vi "ep_Input Power Method.vi"(6 "total input active power [W]":dbl, 8 "error in (no error)":errorcluster, 9 "nameplate information":T1, 11 "efficiency values [%]":dbl[](array[numeric])) -> (0 "error out":errorcluster, 2 "efficiency [%]":dbl, 3 "load [W]":dbl)   [LabVIEW 2014, in "NI_EP_Motor Monitoring.lvlib"]
uses:
  <vilib>/addons/Electrical Power/Motor Monitoring/NI_EP_Motor Monitoring.lvlib
  <vilib>/addons/Electrical Power/Motor Monitoring/subVIs/ep_Input Power Algorithm.ctl
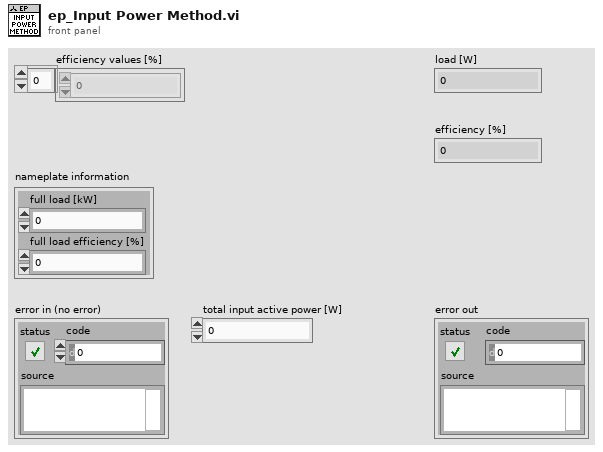
[diagram p1: front panel]
types:
  T1 = cluster{"full load [kW]":dbl, "full load efficiency [%]":dbl}
  T2 = typedef "NI_EP_Motor Monitoring.lvlib/ep_Input Power Algorithm.ctl" = enum16{"interpolate eff.", "use min eff.", "use default eff."}
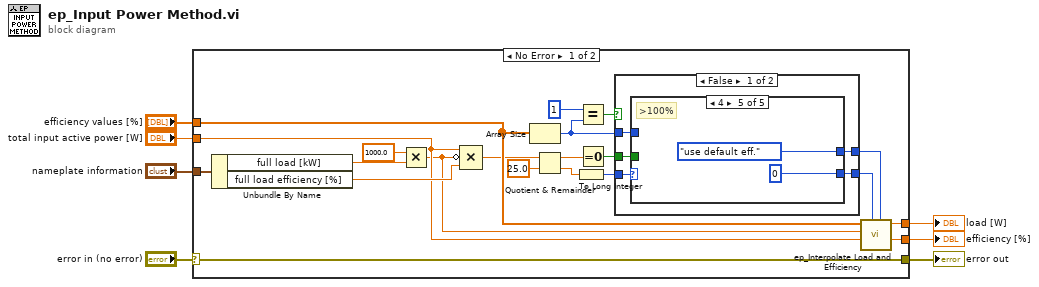
[diagram p0: block diagram]
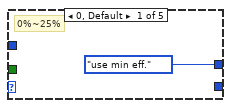
[diagram p2: hidden frame]
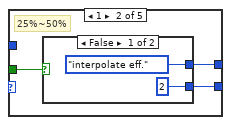
[diagram p3: hidden frame]
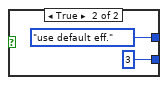
[diagram p4: hidden frame]
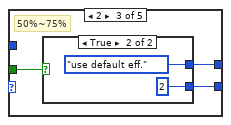
[diagram p5: hidden frame]
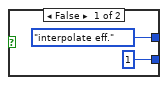
[diagram p6: hidden frame]
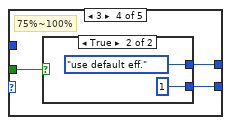
[diagram p7: hidden frame]
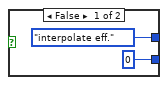
[diagram p8: hidden frame]
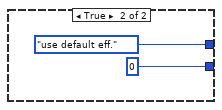
[diagram p9: hidden frame]
diagram:
  n1 = case shown="No Error" "error in (no error)" {
    selector: "error in (no error)" -> [w28 w60]
    tunnel: "efficiency values [%]" -> [w20 _]
    tunnel: "nameplate information" -> [w27 _]
    tunnel: "total input active power [W]" -> [w12 _]
    tunnel: [w28 w60] -> w3
    tunnel: [w26 _] -> w2
    tunnel: [w11 _] -> w1
    frame No Error {
      n2 = Unbundle By Name(w27) -> ("full load [kW]"=w9:dbl, "full load efficiency [%]"=w19:dbl)
      n3 = Multiply(x=1000.0, y=w9) -> (x*y=w10:dbl)
      n4 = Compound Arithmetic op=MULTIPLY(w12, invert w10, w19) -> (w15:dbl)
      n5 = Array Size(array=w20) -> (size(s)=w23:i32)
      n6 = Quotient & Remainder(x=w15, y=25.0) -> (x-y*floor(x/y)=w14:dbl, floor(x/y)=w17:dbl)
      n7 = To Long Integer(number=w17) -> (32bit integer=w25:i32)
      n8 = Equal?(x=1, y=w23) -> (x = y?=w24:bool)
      n9 = Equal To 0?(x=w14) -> (x = 0?=w13:bool)
      n10 = case shown="False" w24 {
        tunnel: w25 -> [w33 _]
        tunnel: [w32 ep_Input_Power_Algorithm."use default eff." ("algorithm")] -> w21
        tunnel: [w31 0] -> w22
        tunnel: w23 -> [w30 _]
        tunnel: w13 -> [w29 _]
        frame False {
          n11 = case shown="4" w33 {
            tunnel: [ep_Input_Power_Algorithm."use min eff." ("algorithm") w37 w44 w51 ep_Input_Power_Algorithm."use default eff." ("algorithm")] -> w32
            tunnel: [_ w36 w43 w50 0] -> w31
            tunnel: w30 -> [_ _ _ _ _]
            tunnel: w29 -> [_ w35 w42 w49 _]
            frame 0, Default {
              # "0%~25%"
            }
            frame 1 {
              # "25%~50%"
              n12 = case shown="False" w35 {
                tunnel: [ep_Input_Power_Algorithm."interpolate eff." ("algorithm") ep_Input_Power_Algorithm."use default eff." ("algorithm")] -> w37
                tunnel: [2 3] -> w36
                frame False {
                }
                frame True {
                }
              }
            }
            frame 2 {
              # "50%~75%"
              n13 = case shown="True" w42 {
                tunnel: [ep_Input_Power_Algorithm."interpolate eff." ("algorithm") ep_Input_Power_Algorithm."use default eff." ("algorithm")] -> w44
                tunnel: [1 2] -> w43
                frame False {
                }
                frame True {
                }
              }
            }
            frame 3 {
              # "75%~100%"
              n14 = case shown="True" w49 {
                tunnel: [ep_Input_Power_Algorithm."interpolate eff." ("algorithm") ep_Input_Power_Algorithm."use default eff." ("algorithm")] -> w51
                tunnel: [0 1] -> w50
                frame False {
                }
                frame True {
                }
              }
            }
            frame 4 {
              # ">100%"
            }
          }
        }
        frame True {
        }
      }
      n15 = call <vilib>:"ep_Interpolate Load and Efficiency.vi"("algorithm"=w21, "index"=w22, "total input active power [W]"=w12, "full load [W]"=w10, "efficiency values [%]"=w20) -> ("efficiency [%]"=w11:dbl, "load [W]"=w26:dbl)  [unwired: 5 in]
    }
    frame Error {
    }
  }
  "error out" <- w3
  "load [W]" <- w2
  "efficiency [%]" <- w1
